vi "AddRootName.vi"(9 "ItemTags":string[](array[string]), 10 "Ident":i32[](array[numeric]), 11 "ItemNames":string[](array[string])) -> (1 "ItemIdents":i32[](array[numeric]), 2 "ChildTags":string[](array[string]), 3 "LeftCellStrings":string[](array[string]))   [LabVIEW 2016, in "Folder_Mgmt.lvclass"]
uses:
  Folder_Mgmt.lvclass
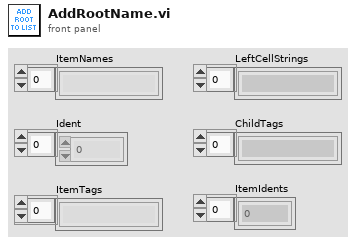
[diagram p1: front panel]
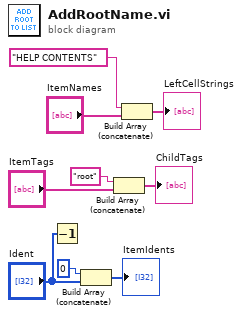
[diagram p0: block diagram]
diagram:
  n1 = Decrement(x="Ident") -> ()  [unwired: 1 out]
  n2 = Build Array (concatenate)(0 ("Numeric"), "Ident") -> (→"ItemIdents":i32[])
  n3 = Build Array (concatenate)("root", "ItemTags") -> (→"ChildTags":string[])
  n4 = Build Array (concatenate)("HELP CONTENTS" ("String"), "ItemNames") -> (→"LeftCellStrings":string[])
